vi "UMM_Edict.vi"(10 "信息":string[](array[string])) -> (2 "信息 out":string[](array[string]), 3 "sure？":bool)   [LabVIEW 2019, in "User Management Model.lvclass"]
uses:
  User Management Model.lvclass
panel:
  in  "权限:":string(combo) caption="Combo Box"
  in  "cancel":bool
  in  "yes":bool=TRUE
  in  "登陆名:":string caption="String"
  in  "密码:":string caption="String"
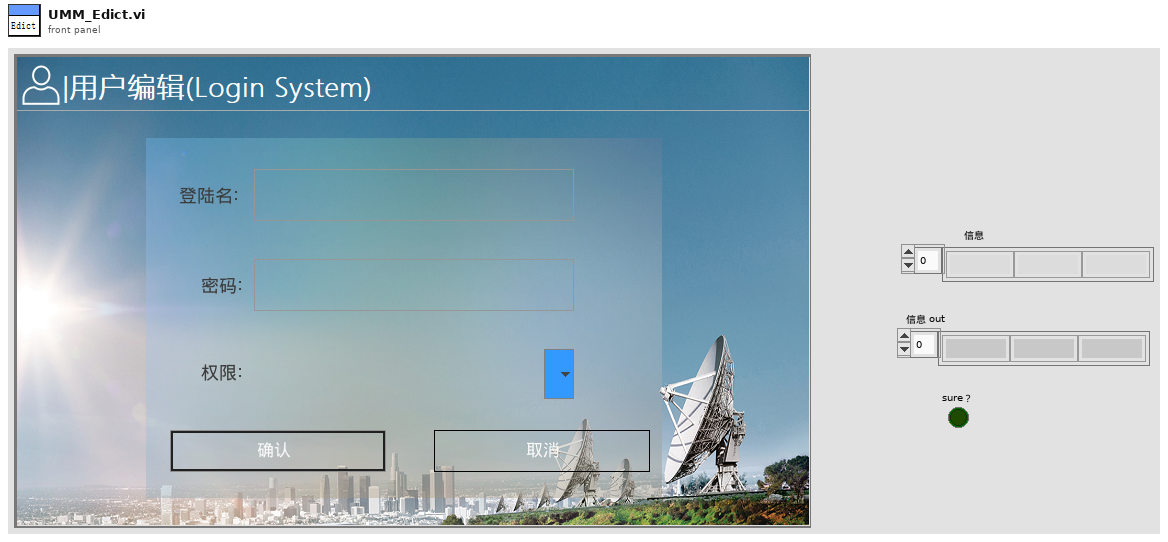
[diagram p1: front panel]
types:
  T1 = enum32{"Invalid", "Standard", "Closed", "Hidden", "Minimized", "Maximized"}
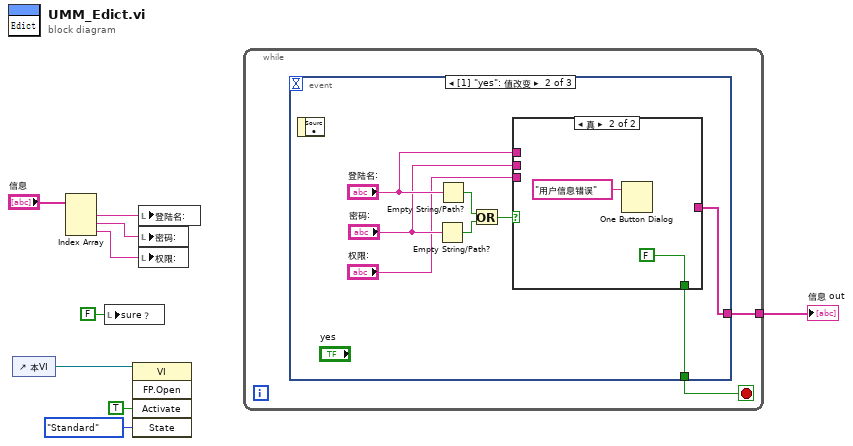
[diagram p0: block diagram]
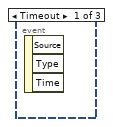
[diagram p2: hidden frame]
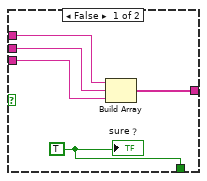
[diagram p3: hidden frame]
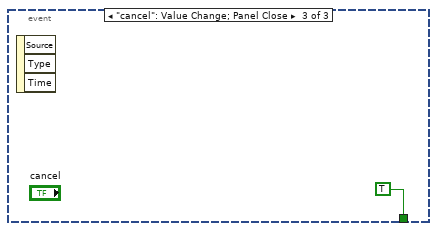
[diagram p4: hidden frame]
diagram:
  n1 = control-ref of="本VI"() -> (w3:refnum<vi>)
  n2 = Index Array(array="信息") -> (element #1=w8:string, element #2=w7:string, element #3=w6:string)  [unwired: 3 in]
  n3 = local write "sure？"(FALSE ("sure？")) -> ()
  n4 = invoke class="VI" method="FP.Open"(reference=w3, "Activate"=TRUE ("激活？"), "State"=T1."Standard" ("状态")) -> ()  [unwired: 2 in, 5 out]
  n5 = local write "登陆名:"(w8) -> ()
  n6 = local write "密码:"(w7) -> ()
  n7 = local write "权限:"(w6) -> ()
  n8 = while {
    tunnel: [w11] -> w5
    stop <- w10 stop-if-true
    n9 = event shown="[1] \"yes\": 值改变" {
      selector: _ -> [_ _ _]
      dyn-events: _ -> [_ _ _]
      timeout: _ -> [_ _ _]
      tunnel: [_ w13 _] -> w11
      tunnel: [_ w12 TRUE] -> w10
      event Timeout {
        n10 = event-data() -> ()  [unwired: 1 in, 3 out]
      }
      event "yes": Value Change {
        n11 = event-data() -> ()  [unwired: 1 in, 1 out]
        n12 = Empty String/Path?(string/path="密码:") -> (empty?=w18:bool)
        n13 = Empty String/Path?(string/path="登陆名:") -> (empty?=w19:bool)
        n14 = Or(x=w19, y=w18) -> (x .or. y?=w17:bool)
        n15 = case shown="真" w17 {
          tunnel: "登陆名:" -> [w24 _]
          tunnel: "密码:" -> [w23 _]
          tunnel: "权限:" -> [w22 _]
          tunnel: [w21 _] -> w13
          tunnel: [w20 FALSE] -> w12
          frame False {
            w20 = TRUE
            n16 = Build Array(w24, w23, w22) -> (w21:string[])
            "sure？" <- w20
          }
          frame True {
            n17 = One Button Dialog(message="用户信息错误" ("消息")) -> ()  [unwired: 1 in, 1 out]
          }
        }
      }
      event "cancel": Value Change; Panel Close {
        n18 = event-data() -> ()  [unwired: 1 in, 3 out]
      }
    }
  }
  "信息 out" <- w5
